vi "Adaptive.vi"() -> ()   [LabVIEW 2017]
doc: "The myRIO Project template acquires acceleration data from the onboard accelerometer and displays the changes of acceleration values in a waveform chart."
uses:
  <vilib>/myRIO/Instrument Drivers/Onboard IO/DIO/typedefs/DIO Reference.ctl
  <vilib>/myRIO/Common/Instrument Driver Framework/Utilities/typedefs/myRIO Generic Hardware Reference.ctl
  <vilib>/myRIO/Common/Instrument Driver Framework/Utilities/typedefs/Hardware Version Enum.ctl
  <vilib>/myRIO/Common/Instrument Driver Framework/Utilities/typedefs/myRIO v1.0 Reference.ctl
  <vilib>/myRIO/Common/Instrument Driver Framework/Utilities/typedefs/Generic FPGA Reference.ctl
  <vilib>/myRIO/Common/Instrument Driver Framework/myRIO v1.0/DIO/typedefs/DIO Channels List.ctl
  <vilib>/myRIO/Common/Instrument Driver Framework/myRIO v1.0/DIO/typedefs/DIO Channels Enum.ctl
  <vilib>/userdefined/High Color/nirio_resource_hc.ctl
  <vilib>/Platform/TimedLoop/XDataNode/timing_clust.ctl
  <vilib>/Platform/TimedLoop/XDataNode/nitl_modes.ctl
  <vilib>/Platform/TimedLoop/XDataNode/wakeup.ctl
  <vilib>/myRIO/Common/Instrument Driver Framework/myRIO v1.0/Encoder/typedefs/Encoder Signal Mode.ctl
  <vilib>/myRIO/Instrument Drivers/Onboard IO/Encoder/typedefs/Encoder Reference.ctl
  <vilib>/myRIO/Common/Instrument Driver Framework/myRIO v1.0/Encoder/typedefs/Encoder Channels Enum.ctl
  <vilib>/myRIO/Common/Instrument Driver Framework/myRIO v1.0/Encoder/typedefs/Encoder Configuration v1.0.ctl
  <vilib>/myRIO/Instrument Drivers/Onboard IO/AI/typedefs/AI Reference.ctl
  <vilib>/myRIO/Common/Instrument Driver Framework/myRIO v1.0/AI/typedefs/AI Channels List.ctl
  <vilib>/myRIO/Common/Instrument Driver Framework/myRIO v1.0/AI/typedefs/AI Channels Enum.ctl
  <vilib>/myRIO/Common/Instrument Driver Framework/Utilities/typedefs/Analog Scaling Constants List.ctl
  <vilib>/myRIO/Common/Instrument Driver Framework/Utilities/typedefs/Analog Scaling Constants.ctl
  <vilib>/myRIO/Instrument Drivers/Onboard IO/PWM/typedefs/PWM Reference.ctl
  <vilib>/myRIO/Common/Instrument Driver Framework/myRIO v1.0/PWM/typedefs/PWM Channels Enum.ctl
  <vilib>/myRIO/Instrument Drivers/Onboard IO/PWM/typedefs/PWM Configuration.ctl
  <vilib>/myRIO/Common/Instrument Driver Framework/Utilities/vis/Is FPGA Ref Available.vi
  <vilib>/myRIO/Common/Instrument Driver Framework/myRIO v1.0/DIO/vis/myRIO v1.1 Open DIO.vi
  <vilib>/myRIO/Instrument Drivers/Onboard IO/DIO/vis/Write.vi
  <vilib>/myRIO/Common/Instrument Driver Framework/myRIO v1.0/AI/vis/myRIO v1.1 Open AI.vi
  <vilib>/myRIO/Instrument Drivers/Onboard IO/AI/vis/Read.vi
  <vilib>/myRIO/Common/Instrument Driver Framework/myRIO v1.0/Encoder/vis/myRIO v1.1 Open Encoder.vi
  <vilib>/myRIO/Instrument Drivers/Onboard IO/Encoder/vis/Read.vi
  <vilib>/myRIO/Common/Instrument Driver Framework/myRIO v1.0/PWM/vis/myRIO v1.1 Open PWM.vi
  <vilib>/myRIO/Instrument Drivers/Onboard IO/PWM/vis/Set Duty Cycle and Frequency.vi
  <vilib>/myRIO/Common/Instrument Driver Framework/Utilities/vis/Validate Channels.vi
  <vilib>/myRIO/Common/Instrument Driver Framework/myRIO v1.0/DIO/vis/myRIO v1.0 Reserve DIO.vi
  <vilib>/myRIO/Common/Instrument Driver Framework/myRIO v1.0/AI/vis/myRIO v1.0 Reserve AI.vi
  <vilib>/myRIO/Common/Instrument Driver Framework/myRIO v1.0/Encoder/vis/myRIO v1.0 Reserve Encoder.vi
  <vilib>/myRIO/Common/Instrument Driver Framework/myRIO v1.0/PWM/vis/myRIO v1.0 Reserve PWM.vi
  <vilib>/myRIO/Common/Instrument Driver Framework/myRIO v1.0/Resource Manager/vis/myRIO v1.0 Reserve Channel List.vi
  <vilib>/myRIO/Common/Instrument Driver Framework/myRIO v1.0/DIO/vis/myRIO v1.0 Build MUX Configuration DIO.vi
  <vilib>/myRIO/Common/Instrument Driver Framework/myRIO v1.0/AI/vis/myRIO v1.0 Build MUX Configuration AI.vi
  <vilib>/myRIO/Common/Instrument Driver Framework/myRIO v1.0/Encoder/vis/myRIO v1.0 Build MUX Configuration Encoder.vi
  <vilib>/myRIO/Common/Instrument Driver Framework/myRIO v1.0/PWM/vis/myRIO v1.0 Build MUX Configuration PWM.vi
  <vilib>/myRIO/Common/Instrument Driver Framework/myRIO v1.0/Resource Manager/vis/myRIO v1.0 Reserve Channel.vi
  <vilib>/myRIO/Common/Instrument Driver Framework/myRIO v1.0/Resource Manager/vis/myRIO v1.0 Unreserve Channel.vi
  <vilib>/myRIO/Common/Instrument Driver Framework/myRIO v1.0/Resource Manager/vis/myRIO v1.0 Create Configuration List.vi
  <vilib>/myRIO/Common/Instrument Driver Framework/myRIO v1.0/Resource Manager/vis/myRIO v1.0 Build Mutex Name.vi
  <vilib>/Utility/VariantDataType/GetNumericInfo.vi
  <vilib>/Utility/error.llb/Error Cluster From Error Code.vi
  <vilib>/myRIO/Common/Instrument Driver Framework/myRIO v1.0/myRIO v1.1 Open.vi
  <vilib>/myRIO/Common/Instrument Driver Framework/Utilities/vis/IO Manager.vi
  <vilib>/myRIO/Common/Instrument Driver Framework/Utilities/vis/Configuration Manager.vi
  <vilib>/myRIO/Common/Instrument Driver Framework/myRIO v1.0/Resource Manager/vis/myRIO v1.0 Configure IO.vi
  <vilib>/myRIO/Common/Instrument Driver Framework/myRIO v1.0/myRIO v1.0 Close.vi
  <vilib>/myRIO/Common/Instrument Driver Framework/myRIO v1.0/DIO/vis/myRIO v1.0 Write DIO.vi
  <vilib>/myRIO/Common/Instrument Driver Framework/myRIO v1.0/Encoder/vis/myRIO v1.0 Configure Encoder.vi
  <vilib>/myRIO/Common/Instrument Driver Framework/myRIO v1.0/Encoder/vis/myRIO v1.0 Read Encoder.vi
  <vilib>/myRIO/Common/Instrument Driver Framework/myRIO v1.0/AI/vis/myRIO v1.0 Get Scaling Constants AI.vi
  <vilib>/myRIO/Common/Instrument Driver Framework/myRIO v1.0/AI/vis/myRIO v1.0 Read AI.vi
  <vilib>/myRIO/Common/Instrument Driver Framework/myRIO v1.0/PWM/vis/myRIO v1.0 Write PWM.vi
  <vilib>/myRIO/Express VI/Onboard IO/DO/DO Express VI.xnode
  <vilib>/myRIO/Instrument Drivers/Onboard IO/DIO/vis/myRIO DIO Open.xnode
  <vilib>/platform/TimedLoop/XDataNode/XDataNode.xnode
  <vilib>/myRIO/Express VI/Onboard IO/Encoder/Encoder Express VI.xnode
  <vilib>/myRIO/Instrument Drivers/Onboard IO/Encoder/vis/myRIO Encoder Open.xnode
  <vilib>/myRIO/Express VI/Onboard IO/AI/AI Express VI.xnode
  <vilib>/myRIO/Instrument Drivers/Onboard IO/AI/vis/myRIO AI Open.xnode
  <vilib>/myRIO/Express VI/Onboard IO/PWM/PWM Express VI.xnode
  <vilib>/myRIO/Instrument Drivers/Onboard IO/PWM/vis/myRIO PWM Open.xnode
  <vilib>/myRIO/Instrument Drivers/Onboard IO/DIO/DIO.lvlib
  <vilib>/myRIO/Instrument Drivers/Onboard IO/PWM/PWM.lvlib
  <vilib>/myRIO/Instrument Drivers/Onboard IO/AI/AI.lvlib
  <vilib>/myRIO/Instrument Drivers/Onboard IO/Encoder/Encoder.lvlib
  <vilib>/Platform/TimedLoop/XDataNode/XDNodeRunTimeDep.lvlib
panel:
  out "T":dbl(graph)
  out "Tempo":dbl
  in  "LIMin":dbl=15.0 min=0.0 step=0.1
  out "dt":dbl
  in  "Zerar Rede Neural":bool
  out "Aceleração da Ponta":dbl(graph)
  out "accp":dbl
  out "thpp":dbl
  out "thp":dbl
  out "Thetapp":cluster{"Thetapp":dbl, "thppD":dbl}(graph)
  out "Thetap":cluster{"Thetap":dbl, "thpD":dbl}(graph)
  out "Theta":cluster{"Theta":dbl, "thD":dbl}(graph)
  out "th":dbl
  in  "srpC":dbl=60.0 min=1.0 step=1.0
  in  "kIN":dbl=20.0 min=1.0 step=1.0
  in  "phiIN":dbl=15.0 step=0.1
  in  "apIN":dbl=1.8 min=0.0 step=0.1
  in  "Min":dbl=100.0 min=1.0 step=1.0
  in  "Funcionamento":bool
  in  "Lambda":dbl=15.0 min=0.0 max=10000.0 step=0.1
  in  "Tab Control":T1(tab)
  in  "Posicao Angular":dbl(knob) min=-45.0 max=45.0 step=5.0 scale=45.0..-45.0
  in  "Amplitude":dbl(knob)=45.0 min=0.0 max=45.0 step=1.0 scale=0.0..45.0
  in  "Frequencia (Hz)":dbl(knob)=0.10000000000000002 min=0.0 max=3.0 step=0.1 scale=0.0..3.0
  in  "Amplitude":dbl(knob)=45.0 min=0.0 max=45.0 step=1.0 scale=0.0..45.0
  in  "Frequencia (Hz)":dbl(knob)=0.10000000000000002 min=0.0 max=3.0 step=0.1 scale=0.0..3.0
  in  "Período":dbl(knob)=2.5 min=1.5 max=10.0 step=0.5 scale=1.5..10.0
  in  "Reducao de vibração":bool=TRUE
  in  "Ciclo de Controle":bool
  out "th(°)":dbl
  in  "Zerar contador":bool
  in  "Ciclo de aquisição":bool
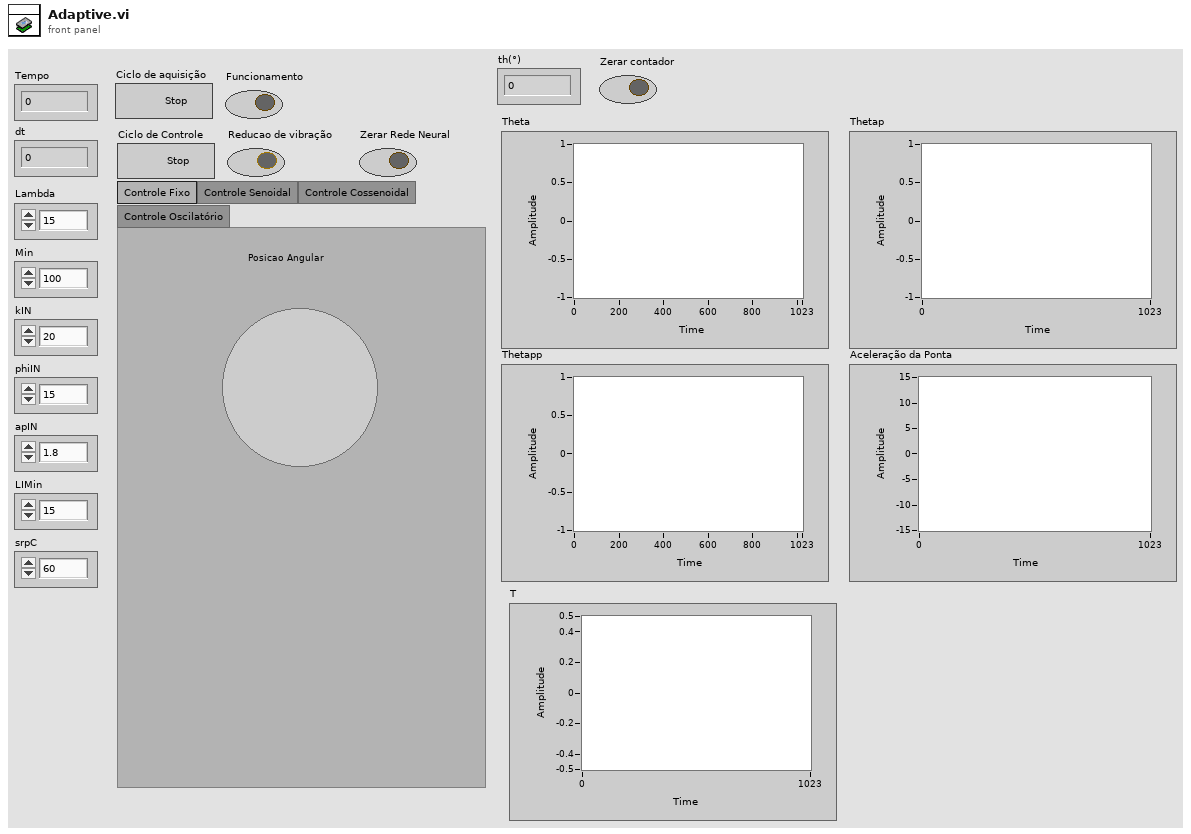
[diagram p1: front panel]
types:
  T1 = enum32{"Controle Fixo", "Controle Senoidal", "Controle Cossenoidal", "Controle Oscilatório"}
  T2 = enum16{"open", "replace", "create", "open or create", "replace or create", "replace or create with confirmation"}
  T3 = typedef "DIO.lvlib/DIO Reference.ctl" = cluster{"myRIO Reference":T4, "DIO Channels List":T8}
  T4 = typedef "myRIO Generic Hardware Reference.ctl" = cluster{"myRIO Model":T5, "myRIO Hardware Reference":T6}
  T5 = typedef "Hardware Version Enum.ctl" = enum16{"Unknown", "myRIO-1900", "myRIO-1950", "roboRIO", "NI ELVIS RIO CM"}
  T6 = typedef "myRIO v1.0 Reference.ctl" = cluster{"Generic FPGA Reference":T7, "Allow multiple opens":bool}
  T7 = typedef "Generic FPGA Reference.ctl" = refnum<k20>
  T8 = typedef "DIO Channels List.ctl" = T9[]
  T9 = typedef "DIO Channels Enum.ctl" = enum16{"Not Connected", "C/DIO0", "C/DIO1", "C/DIO2", "C/DIO3", "C/DIO4", "C/DIO5", "C/DIO6", "C/DIO7", "A/DIO0", "A/DIO1", "A/DIO2", "A/DIO3", "A/DIO4", "A/DIO5", "A/DIO6", "A/DIO7", "A/DIO8", "A/DIO9", "A/DIO10", "A/DIO11", "A/DIO12", "A/DIO13", "A/DIO14", "A/DIO15", "B/DIO0", "B/DIO1", "B/DIO2", "B/DIO3", "B/DIO4", "B/DIO5", "B/DIO6", "B/DIO7", "B/DIO8", "B/DIO9", "B/DIO10", "B/DIO11", "B/DIO12", "B/DIO13", "B/DIO14", "B/DIO15", "LED0", "LED1", "LED2", "LED3", "Button0", "DIO/DIO0", "DIO/DIO1", "DIO/DIO2", "DIO/DIO3", "DIO/DIO4", "DIO/DIO5", "DIO/DIO6", "DIO/DIO7", "DIO/DIO8", "DIO/DIO9", "SPI/CS0", "SPI/CS1", "SPI/CS2", "SPI/CS3", "LED RADIO (Green)", "LED RADIO (Red)", "LED COMM (Green)", "LED COMM (Red)", "LED MODE (Green)", "LED MODE (Red)"}
  T10 = typedef "nirio_resource_hc.ctl" = tag
  T11 = typedef "XDNodeRunTimeDep.lvlib/timing_clust.ctl" = cluster{"Expected End [f-1]":u64, "Actual End [f-1]":u64, "Finished Late? [f-1]":bool, "Expected End [i-1]":u64, "Actual End [i-1]":u64, "Finished Late? [i-1]":bool, "Expected Start [i]":u64, "Actual Start [i]":u64, "Expected Start [f]":u64, "Actual Start [f]":u64, "Source Name":string, "Structure Name":string, "Period":i64, "Deadline":i64, "Offset":i64, "Start":i64, "Priority":i32, "Timeout":i32, "Mode":T12, "Wakeup Reason":T13, "Error":errorcluster, "Source Type":string, "Secondary Source Type":string, "Global End Time":u64, "Global Start Time":u64, "Frame Duration":u64, "Iteration Duration":u64, "Assigned CPU":i32, "I/O Scan Engine Mode":u32}
  T12 = typedef "XDNodeRunTimeDep.lvlib/nitl_modes.ctl" = enum32{"No Change", "Process missed periods, maintain original phase", "Discard missed periods, maintain original phase", "Process missed periods, ignore original phase", "Discard missed periods, ignore original phase"}
  T13 = typedef "XDNodeRunTimeDep.lvlib/wakeup.ctl" = enum32{"Normal", "Aborted", "Asynchronous wakeup", "Timing source error", "Timed loop error", "Timeout"}
  T14 = typedef "Encoder.lvlib/Encoder Reference.ctl" = cluster{"myRIO Reference":T4, "Encoder Channels Enum":T15}
  T15 = typedef "Encoder Channels Enum.ctl" = enum16{"Not Connected", "C/ENC0", "C/ENC1", "A/ENC", "B/ENC", "DIO/ENC0", "DIO/ENC1", "DIO/ENC2", "DIO/ENC3", "DIO/ENC4"}
  T16 = typedef "Encoder Signal Mode.ctl" = enum16{"Quadrature phase signal", "Step and direction signal"}
  T17 = typedef "AI.lvlib/AI Reference.ctl" = cluster{"myRIO Reference":T4, "AI Channels List":T18, "AI Scaling Constants List":T20}
  T18 = typedef "AI Channels List.ctl" = T19[]
  T19 = typedef "AI Channels Enum.ctl" = enum16{"Not Connected", "AudioIn/Left", "AudioIn/Right", "C/AI0", "C/AI1", "A/AI0", "A/AI1", "A/AI2", "A/AI3", "B/AI0", "B/AI1", "B/AI2", "B/AI3", "AI/AI0", "AI/AI1", "AI/AI2", "AI/AI3"}
  T20 = typedef "Analog Scaling Constants List.ctl" = T21[]
  T21 = typedef "Analog Scaling Constants.ctl" = cluster{"LSB Weight (Volts)":dbl, "Offset (Volts)":dbl, "Signed?":bool}
  T22 = typedef "PWM.lvlib/PWM Reference.ctl" = cluster{"myRIO Reference":T4, "PWM Channels Enum":T23, "PWM Configuration":T24}
  T23 = typedef "PWM Channels Enum.ctl" = enum16{"Not Connected", "C/PWM0", "C/PWM1", "A/PWM0", "A/PWM1", "A/PWM2", "B/PWM0", "B/PWM1", "B/PWM2", "PWM/PWM0", "PWM/PWM1", "PWM/PWM2", "PWM/PWM3", "PWM/PWM4", "PWM/PWM5", "PWM/PWM6", "PWM/PWM7", "PWM/PWM8", "PWM/PWM9"}
  T24 = typedef "PWM.lvlib/PWM Configuration.ctl" = cluster{"Frequency":dbl, "Duty Cycle":dbl}
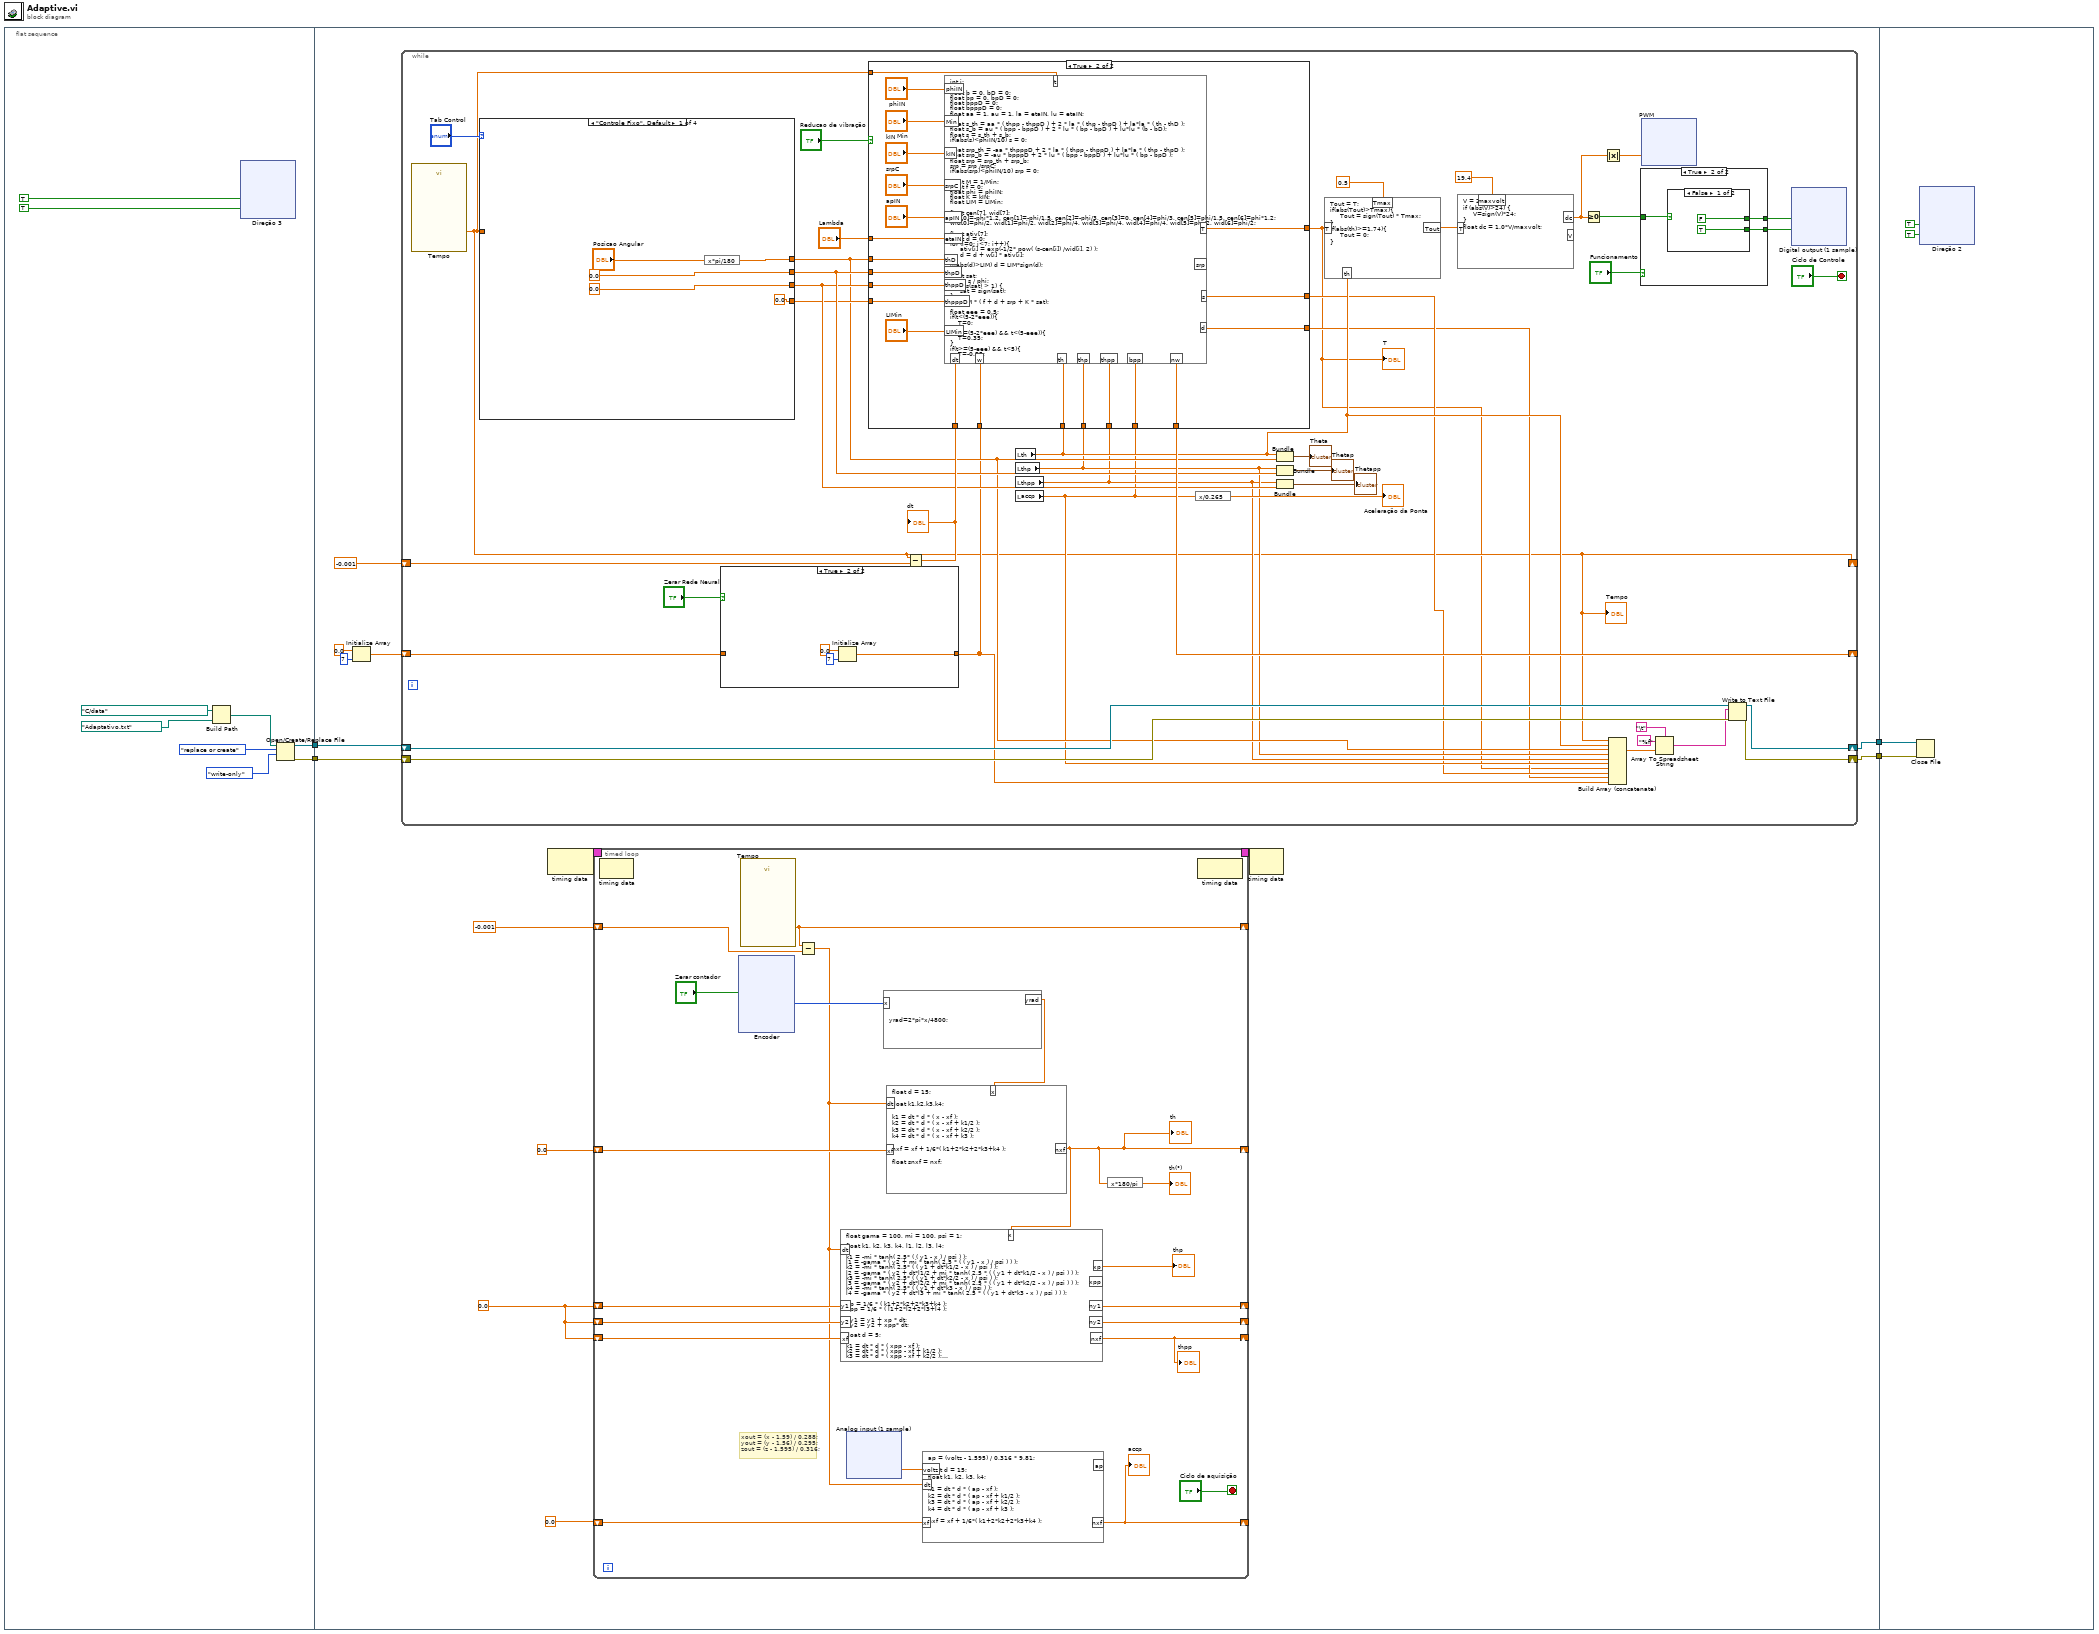
[diagram p0: block diagram]
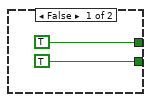
[diagram p2: hidden frame]
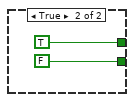
[diagram p3: hidden frame]
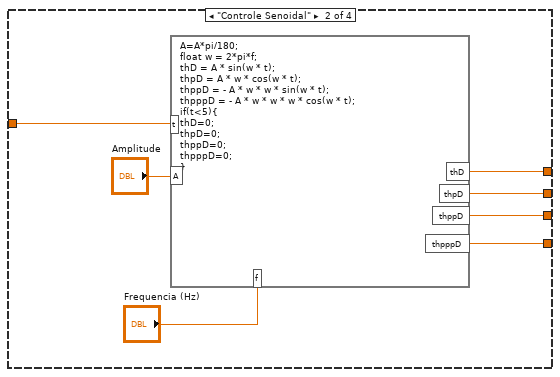
[diagram p4: hidden frame]
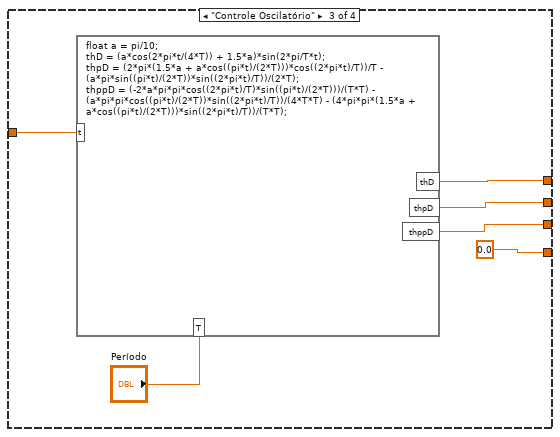
[diagram p5: hidden frame]
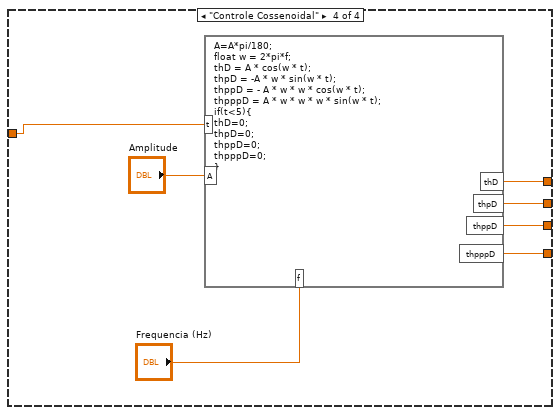
[diagram p6: hidden frame]
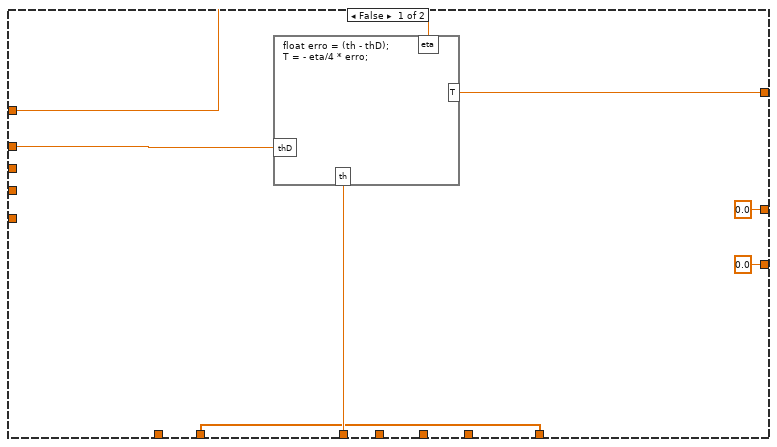
[diagram p7: hidden frame]
diagram:
  n1 = flat-sequence {
    tunnel: [w6] -> w4
    tunnel: [w5] -> w2
    tunnel: w4 -> [w53]
    tunnel: [w52] -> w3
    tunnel: w2 -> [w50]
    tunnel: [w51] -> w1
    tunnel: w3 -> [w353]
    tunnel: w1 -> [w352]
    frame #0 {
      n2 = Build Path(base path=path "C:/data", name or relative path=path "Adaptativo.txt") -> (appended path=w9:path)
      n3 = xnode "Direção 3"("In1 (A/DIO8 (Pin 27))"=TRUE, "In2 (A/DIO9 (Pin 29))"=TRUE) -> ()  [unwired: 1 in, 1 out]
      n4 = Open/Create/Replace File(file path (use dialog)=w9, operation (0:open)=T2."replace or create", access (0:read/write)=enum16{"read/write", "read-only", "write-only"}."write-only") -> (refnum out=w6:refnum<file>, error out=w5:errorcluster)  [unwired: 3 in, 1 out]
    }
    frame #1 {
      w60 = 0.0
      n5 = Initialize Array(0.0 ("element"), 7 ("dimension size")) -> (w58:dbl[])
      n6 = while {
        shift-right: [w206] -> _
        shift-left: w58 -> [w192]
        shift-right: [w175] -> _
        shift-left: -0.001 ("element") -> [w205]
        shift-right: [w187] -> w52
        shift-left: w53 -> [w186]
        shift-right: [w185] -> w51
        shift-left: w50 -> [w184]
        stop <- "Ciclo de Controle" stop-if-true
        n7 = call "Tempo"() -> ("Elapsed Time (s)"=w175:dbl)  [unwired: 12 in, 7 out]
        "Tempo" <- w175
        n8 = case shown="\"Controle Fixo\", Default" "Tab Control" {
          tunnel: [w224 w233 w237 w243] -> w182
          tunnel: w175 -> [_ w232 w235 w244]
          tunnel: [0.0 w229 w238 w242] -> w198
          tunnel: [0.0 w228 w239 w241] -> w197
          tunnel: [0.0 ("thpppD") w227 0.0 ("thpppD") w240] -> w189
          frame "Controle Fixo", Default {
            n9 = expression code="x*pi/180"("Posicao Angular") -> (w224:dbl)
          }
          frame "Controle Senoidal" {
            n10 = formula code="A=A*pi/180;\nfloat w = 2*pi*f;\nthD = A * sin(w * t);\nthpD = A * w * cos(w * t);\nthppD = - A * w * w * sin(w * t);\nthpppD = - A * w * w * w * cos(w * t);\nif(t<5){\nthD=0;\nthpD=0;\nthppD=0;\nthpppD=0;\n}"("t"=w232, "A"="Amplitude", "f"="Frequencia (Hz)") -> ("thD"=w233:dbl, "thpD"=w229:dbl, "thppD"=w228:dbl, "thpppD"=w227:dbl)
          }
          frame "Controle Oscilatório" {
            n11 = formula code="float a = pi/10;\nthD = (a*cos(2*pi*t/(4*T)) + 1.5*a)*sin(2*pi/T*t);\nthpD = (2*pi*(1.5*a + a*cos((pi*t)/(2*T)))*cos((2*pi*t)/T))/T - (a*pi*sin((pi*t)/(2*T))*sin((2*pi*t)/T))/(2*T);\nthppD = (-2*a*pi*pi*cos((2*pi*t)/T)*sin((pi*t)/(2*T)))/(T*T) - (a*pi*pi*cos((pi*t)/(2*T))*sin((2*pi*t)/T))/(4*T*T) - (4*pi*pi*(1.5*a + a*cos((pi*t)/(2*T)))*sin((2*pi*t)/T))/(T*T);"("t"=w235, "T"="Período") -> ("thD"=w237:dbl, "thpD"=w238:dbl, "thppD"=w239:dbl)
          }
          frame "Controle Cossenoidal" {
            n12 = formula code="A=A*pi/180;\nfloat w = 2*pi*f;\nthD = A * cos(w * t);\nthpD = -A * w * sin(w * t);\nthppD = - A * w * w * cos(w * t);\nthpppD = A * w * w * w * sin(w * t);\nif(t<5){\nthD=0;\nthpD=0;\nthppD=0;\nthpppD=0;\n}"("t"=w244, "A"="Amplitude", "f"="Frequencia (Hz)") -> ("thD"=w243:dbl, "thpD"=w242:dbl, "thppD"=w241:dbl, "thpppD"=w240:dbl)
          }
        }
        n13 = case shown="True" "Zerar Rede Neural" {
          tunnel: [w347 w348] -> w178
          tunnel: w192 -> [w347 _]
          frame False {
          }
          frame True {
            n14 = Initialize Array(0.0 ("element"), 7 ("dimension size")) -> (w348:dbl[])
          }
        }
        n15 = Subtract(x=w175, y=w205) -> (x-y=w204:dbl)
        "dt" <- w204
        n16 = local read "th"() -> (w183:dbl)
        n17 = local read "thp"() -> (w181:dbl)
        n18 = local read "thpp"() -> (w180:dbl)
        n19 = local read "accp"() -> (w179:dbl)
        n20 = case shown="True" "Reducao de vibração" {
          tunnel: w182 -> [w253 w267]
          tunnel: [w252 w275] -> w170
          tunnel: "Lambda" -> [w251 w274]
          tunnel: [w249 w264] -> w206
          tunnel: w204 -> [_ w273]
          tunnel: w198 -> [_ w266]
          tunnel: w197 -> [_ w265]
          tunnel: w179 -> [_ w263]
          tunnel: w180 -> [_ w262]
          tunnel: w181 -> [_ w261]
          tunnel: w183 -> [w250 w260]
          tunnel: w178 -> [w249 w259]
          tunnel: w189 -> [_ w258]
          tunnel: w175 -> [_ w257]
          tunnel: [0.0 w255] -> w177
          tunnel: [0.0 w254] -> w176
          frame False {
            n21 = formula code="float erro = (th - thD);\nT = - eta/4 * erro;"("thD"=w253, "th"=w250, "eta"=w251) -> ("T"=w252:dbl)
          }
          frame True {
            n22 = formula code="int i;\n\nfloat b = 0, bD = 0;\nfloat bp = 0, bpD = 0;\nfloat bppD = 0;\nfloat bpppD = 0;\nfloat aa = 1, au = 1, la = etaIN, lu = etaIN;\n\nfloat s_th = aa * ( thpp - thppD ) + 2 * la * ( thp - thpD ) + la*la * ( th - thD );\nfloat s_b = au * ( bpp - bppD ) + 2 * lu * ( bp - bpD ) + lu*lu * (b - bD);\nfloat s = s_th + s_b;\nif(abs(s)<phiIN/10) s = 0;\n\nfloat srp_th = -aa * thpppD + 2 * la * ( thpp - thppD ) + la*la * ( thp - thpD );\nfloat srp_b = -au * bpppD + 2 * lu * ( bpp - bppD ) + lu*lu * ( bp - bpD );\nfloat srp = srp_th + srp_b;\nsrp = srp /srpC;\nif(abs(srp)<phiIN/10) srp = 0;\n\nfloat M = 1/Min;\nfloat f = 0;\nfloat phi = phiIN;\nfloat K = kIN;\nfloat LIM = LIMin;\n\nfloat cen[7], wid[7];\ncen[0]=-phi*1.2, cen[1]=-phi/1.5, cen[2]=-phi/3, cen[3]=0, cen[4]=phi/3, cen[5]=phi/1.5, cen[6]=phi*1.2;\nwid[0]=phi/2, wid[1]=phi/2, wid[2]=phi/4, wid[3]=phi/4, wid[4]=phi/4, wid[5]=phi/2, wid[6]=phi/2;\n\nfloat ativ[7];\nfloat d = 0;\nfor (i=0; i<7; i++){\n     ativ[i] = exp(-1/2* pow( (s-cen[i]) /wid[i], 2) );\n     d = d + w[i] * ativ[i];\n}\nif(abs(d)>LIM) d = LIM*sign(d);\n\nfloat sat;\nsat = s / phi;\nif (abs(sat) > 1) {\n     sat = sign(sat);\n}\nT = - M * ( f + d + srp + K * sat);\n\nfloat eee = 0.5;\nif(t<(5-2*eee)){\n    T=0;\n}\nif(t>=(5-2*eee) && t<(5-eee)){\n    T=0.35;\n}\nif(t>=(5-eee) && t<5){\n    T=-0.35;\n}\n\nfloat nw[7];\nfloat ap = apIN;\n/*\n\nif(t<5){\nnw[1]=0;\n}else{\nnw[1]=w[1] + ap * s * dt;\n}\n*/\n\nfor(i=0; i<7; i++){\n    if(t<5){\n        nw[i]=0;\n    }else{\n        nw[i] = w[i] + ap * s * ativ[i] * dt;\n    }\n}"("thD"=w267, "th"=w260, "thp"=w261, "thpp"=w262, "bpp"=w263, "etaIN"=w274, "w"=w259, "dt"=w273, "Min"="Min", "apIN"="apIN", "phiIN"="phiIN", "kIN"="kIN", "srpC"="srpC", "thpD"=w266, "thppD"=w265, "t"=w257, "thpppD"=w258, "LIMin"="LIMin") -> ("T"=w275:dbl, "nw"=w264:dbl[], "s"=w255:dbl, "d"=w254:dbl)  [unwired: 1 out]
          }
        }
        "T" <- w170
        n23 = expression code="x/0.265"(w179) -> (→"Aceleração da Ponta":dbl)
        n24 = Bundle("th"=w183, "thD"=w182) -> (→"Theta":cluster{"th":dbl, "thD":dbl})  [unwired: 1 in]
        n25 = Bundle("thp"=w181, "thpD"=w198) -> (→"Thetap":cluster{"thp":dbl, "thpD":dbl})  [unwired: 1 in]
        n26 = Bundle("thpp"=w180, "thppD"=w197) -> (→"Thetapp":cluster{"thpp":dbl, "thppD":dbl})  [unwired: 1 in]
        n27 = formula code="Tout = T;\nif(abs(Tout)>Tmax){\n     Tout = sign(Tout) * Tmax;\n}\nif(abs(th)>=1.74){\n     Tout = 0;\n}"("Tmax"=0.5 ("input variable"), "T"=w170, "th"=w183) -> ("Tout"=w191:dbl)
        n28 = formula code="V = 24/3*T;\nif (abs(V)>24) {\n     V=sign(V)*24;\n}\nfloat dc = 1.0*V/maxvolt;"("maxvolt"=19.4 ("input variable"), "T"=w191) -> ("dc"=w188:dbl)  [unwired: 1 out]
        n29 = Greater Or Equal To 0?(x=w188) -> (x >= 0?=w203:bool)
        n30 = Absolute Value(x=w188) -> (abs(x)=w211:dbl)
        n31 = Build Array (concatenate)(w175, w183, w182, w181, w180, w179, w170, w177, w176, w178) -> (w172:dbl[])
        n32 = case shown="True" "Funcionamento" {
          tunnel: w203 -> [_ w217]
          tunnel: [TRUE w216] -> w202
          tunnel: [TRUE w215] -> w201
          frame False {
          }
          frame True {
            n33 = case shown="False" w217 {
              tunnel: [FALSE TRUE] -> w216
              tunnel: [TRUE FALSE] -> w215
              frame False {
              }
              frame True {
              }
            }
          }
        }
        n34 = xnode "PWM"("Duty Cycle"=w211) -> ()  [unwired: 1 in, 1 out]
        n35 = Array To Spreadsheet String(delimiter (Tab)="\t", array=w172, 3:"%f" ("format string")) -> (spreadsheet string=w171:string)
        n36 = Write to Text File(file (use dialog)=w186, text=w171, error in=w184) -> (refnum out=w187:refnum<file>, error out=w185:errorcluster)  [unwired: 1 in, 1 out]
        n37 = xnode "Digital output (1 sample)"("In1 (A/DIO8 (Pin 27))"=w202, "In2 (A/DIO9 (Pin 29))"=w201) -> ()  [unwired: 1 in, 1 out]
      }
      n38 = node-c288() -> (w63:T11)  [unwired: 1 in]
      n39 = timed-loop {
        shift-right: [w77] -> _
        shift-left: -0.001 -> [w79]
        shift-right: [w75] -> _
        shift-left: w60 -> [w81]
        shift-right: [w80] -> _
        shift-left: w60 -> [w74]
        shift-right: [w65] -> _
        shift-left: w60 -> [w78]
        timing: w63 -> [_]
        timing-out: [_] -> w62
        shift-right: [w67] -> _
        shift-left: 0.0 -> [w72]
        shift-right: [w64] -> _
        shift-left: 0.0 ("nxf") -> [w69]
        stop <- "Ciclo de aquisição" stop-if-true
        # "xout = (x - 1.59) / 0.288;\nyout = (y - 1.56) / 0.295;\nzout = (z - 1.595) / 0.316;"
        n40 = node-c288() -> ()  [unwired: 1 in, 1 out]
        n41 = xnode "Encoder"("Reset Counter"="Zerar contador") -> ("Counter Value"=w82:i32)  [unwired: 1 in, 3 out]
        n42 = call "Tempo"() -> ("Elapsed Time (s)"=w77:dbl)  [unwired: 12 in, 7 out]
        n43 = Subtract(x=w77, y=w79) -> (x-y=w68:dbl)
        n44 = xnode "Analog input (1 sample)"() -> ("Acc (A/AI2 (Pin 7))"=w76:dbl)  [unwired: 1 in, 1 out]
        n45 = formula code="yrad=2*pi*x/4800;"("x"=w82) -> ("yrad"=w71:dbl)
        n46 = formula code="float d = 15;\n\nfloat k1,k2,k3,k4;\n\nk1 = dt * d * ( x - xf );\nk2 = dt * d * ( x - xf + k1/2 );\nk3 = dt * d * ( x - xf + k2/2 );\nk4 = dt * d * ( x - xf + k3 );\n\nnxf = xf + 1/6*( k1+2*k2+2*k3+k4 );\n\nfloat snxf = nxf;"("x"=w71, "xf"=w72, "dt"=w68) -> ("nxf"=w67:dbl)
        "th" <- w67
        n47 = formula code="float gama = 100, mi = 100, psi = 1;\n\nfloat k1, k2, k3, k4, l1, l2, l3, l4;\n\nk1 = -mi * tanh( 2.5* ( ( y1 - x ) / psi ) );\nl1 = -gama * ( y2 + mi * tanh( 2.5 * ( ( y1 - x ) / psi ) ) );\nk2 = -mi * tanh( 2.5* ( ( y1 + dt*k1/2 - x ) / psi ) );\nl2 = -gama * ( y2 + dt*l1/2 + mi * tanh( 2.5 * ( ( y1 + dt*k1/2 - x ) / psi ) ) );\nk3 = -mi * tanh( 2.5* ( ( y1 + dt*k2/2 - x ) / psi ) );\nl3 = -gama * ( y2 + dt*l2/2 + mi * tanh( 2.5 * ( ( y1 + dt*k2/2 - x ) / psi ) ) );\nk4 = -mi * tanh( 2.5* ( ( y1 + dt*k3 - x ) / psi ) );\nl4 = -gama * ( y2 + dt*l3 + mi * tanh( 2.5 * ( ( y1 + dt*k3 - x ) / psi ) ) );\n\nxp = 1/6 * ( k1+2*k2+2*k3+k4 );\nxpp = 1/6 * ( l1+2*l2+2*l3+l4 );\n\nny1 = y1 + xp * dt;\nny2 = y2 + xpp* dt;\n\nfloat d = 5;\n\nk1 = dt * d * ( xpp - xf );\nk2 = dt * d * ( xpp - xf + k1/2 );\nk3 = dt * d * ( xpp - xf + k2/2 );\nk4 = dt * d * ( xpp - xf + k3 );\n\nnxf = xf + 1/6*( k1+2*k2+2*k3+k4 );"("y1"=w74, "y2"=w81, "x"=w67, "dt"=w68, "xf"=w78) -> ("ny1"=w80:dbl, "ny2"=w75:dbl, "xp"=→"thp":dbl, "nxf"=w65:dbl)  [unwired: 1 out]
        "thpp" <- w65
        n48 = formula code="ap = (voltz - 1.595) / 0.316 * 9.81;\n\nfloat d = 15;\nfloat k1, k2, k3, k4;\n\nk1 = dt * d * ( ap - xf );\nk2 = dt * d * ( ap - xf + k1/2 );\nk3 = dt * d * ( ap - xf + k2/2 );\nk4 = dt * d * ( ap - xf + k3 );\n\nnxf = xf + 1/6*( k1+2*k2+2*k3+k4 );"("voltz"=w76, "dt"=w68, "xf"=w69) -> ("nxf"=w64:dbl)  [unwired: 1 out]
        "accp" <- w64
        n49 = expression code="x*180/pi"(w67) -> (→"th(°)":dbl)
        n50 = node-c288() -> ()  [unwired: 1 in, 1 out]
      }
      n51 = node-c288(w62) -> ()  [unwired: 1 out]
    }
    frame #2 {
      n52 = Close File(refnum=w353, error in=w352) -> ()  [unwired: 2 out]
      n53 = xnode "Direção 2"("In1 (A/DIO8 (Pin 27))"=TRUE, "In2 (A/DIO9 (Pin 29))"=TRUE) -> ()  [unwired: 1 in, 1 out]
    }
  }
